vi "Voltage - Continuous Input.vi"() -> ()   [LabVIEW 2014]
doc: "This example demonstrates how to continuously acquire buffered voltage measurements using a DAQmx device.\n\nFor instructions on how to connect your signals to the DAQ device, refer to your device documentation."
uses:
  <vilib>/DAQmx/configure/task.llb/DAQmx Configure Logging (TDMS).vi
  <vilib>/DAQmx/read.llb/DAQmx Read (Analog 1D Wfm NChan NSamp).vi
  <resource>/objmgr/daqmx.rc
  <vilib>/DAQmx/configure/timing.llb/DAQmx Timing (Sample Clock).vi
  <vilib>/DAQmx/create/channels.llb/DAQmx Create Channel (AI-Voltage-Basic).vi
panel:
  in  "Stop":bool
  out "Waveform Graph":waveform(dbl)[](graph)
  in  "TDMS File Path":path
  in  "Samples per Loop":i32=1000
  in  "Sample Rate":dbl=1000.0
  in  "Sample Clock Source":tag="OnboardClock"
  in  "Terminal Configuration":i32(ring)=-1 items=["default"=-1, "RSE"=10083, "NRSE"=10078, "Differential"=10106, "Pseudodifferential"=12529]
  in  "Max Voltage":dbl=5.0
  in  "Min Voltage":dbl=-5.0
  in  "Physical Channel":tag="Dev1/ai0"
  out "Actual Sample Rate":dbl=1000.0 format="%0.2f"
  in  "Logging Mode":i32(ring)=10231 items=["Off"=10231, "Log and Read"=15842]
  # "Channel Settings"
  # "Acquired Data"
  # "Timing Settings"
  # "Logging Settings"
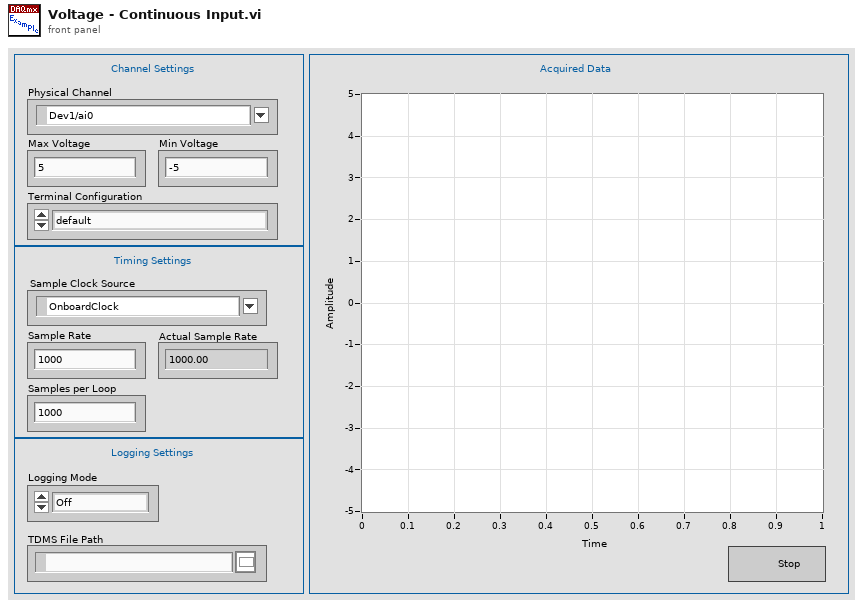
[diagram p1: front panel]
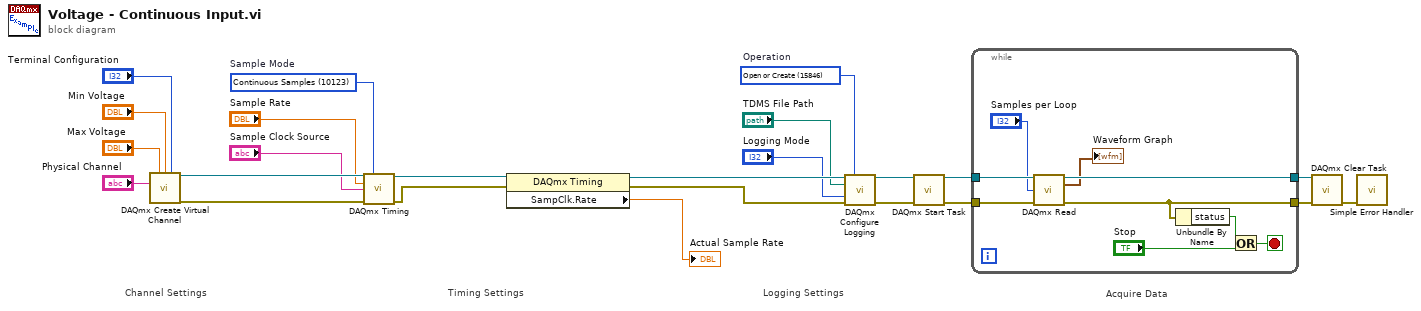
[diagram p0: block diagram]
diagram:
  w17 = 15846 items=["Open"=10437, "Open or Create"=15846, "Create or Replace"=15847, "Create"=15848]  # Operation
  w22 = 10123 items=["Finite Samples"=10178, "Continuous Samples"=10123, "Hardware Timed Single Point"=12522]  # Sample Mode
  # "Acquire Data"
  # "Timing Settings"
  # "Channel Settings"
  # "Logging Settings"
  n1 = call-poly <vilib>:"DAQmx Create Virtual Channel.vi"("maximum value"="Max Voltage", "minimum value"="Min Voltage", "input terminal configuration"="Terminal Configuration", "physical channels"="Physical Channel") -> ("task out"=w20:refnum<k21>, "error out"=w21:errorcluster)  [unwired: 10 in]
  n2 = call-poly <vilib>:"DAQmx Timing.vi"("task/channels in"=w20, "sample mode"=w22, "rate"="Sample Rate", "source"="Sample Clock Source", "error in"=w21) -> ("task out"=w24:refnum<k21>, "error out"=w23:errorcluster)  [unwired: 9 in]
  n3 = property class="DAQmx Timing"(reference=w24, error in=w23) -> (reference out=w19:refnum<k21>, error out=w18:errorcluster, "SampClk.Rate"=→"Actual Sample Rate":dbl)
  n4 = call-poly <vilib>:"DAQmx Configure Logging.vi"("task/channels in"=w19, "operation"=w17, "file path"="TDMS File Path", "logging mode"="Logging Mode", "error in"=w18) -> ("task out"=w2:refnum<k21>, "error out"=w1:errorcluster)  [unwired: 9 in]
  n5 = call <vilib>:"DAQmx Start Task.vi"("task/channels in"=w2, "error in"=w1) -> ("task out"=w16:refnum<k21>, "error out"=w15:errorcluster)  [unwired: 12 in]
  n6 = while {
    tunnel: w16 -> [w33]
    tunnel: w15 -> [w32]
    tunnel: [w29] -> w13
    tunnel: [w30] -> w14
    stop <- w31 stop-if-true
    n7 = call-poly <vilib>:"DAQmx Read.vi"("task/channels in"=w33, "number of samples per channel"="Samples per Loop", "error in"=w32) -> ("task out"=w30:refnum<k21>, "data"=→"Waveform Graph":waveform(dbl)[], "error out"=w29:errorcluster)  [unwired: 10 in]
    n8 = Unbundle By Name(w29) -> ("status"=w28:bool)
    n9 = Or(x=w28, y="Stop") -> (x .or. y?=w31:bool)
  }
  n10 = call <vilib>:"DAQmx Clear Task.vi"("task in"=w14, "error in"=w13) -> ("error out"=w12:errorcluster)  [unwired: 13 in]
  n11 = call <vilib>:"Simple Error Handler.vi"("error in (no error)"=w12) -> ()  [unwired: 4 in, 5 out]
